vi "Handle Transmission.vi"(8 "error in (no error)":errorcluster, 11 "Stuffed Data":string) -> (0 "error out":errorcluster, 2 "Transmission valid?":bool, 3 "Transmission":string)   [LabVIEW 2015, in "LSR Transmission.lvlib"]
uses:
  LSR Transmission.lvlib
panel:
  out "Dropped Frames":i32
  out "Packets Left":i32
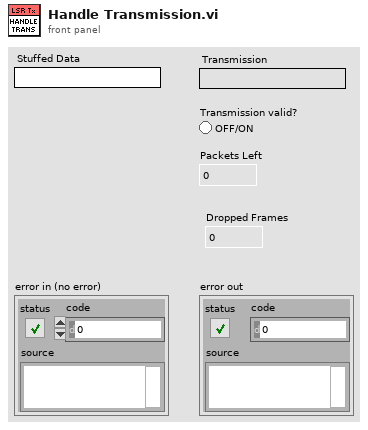
[diagram p1: front panel]
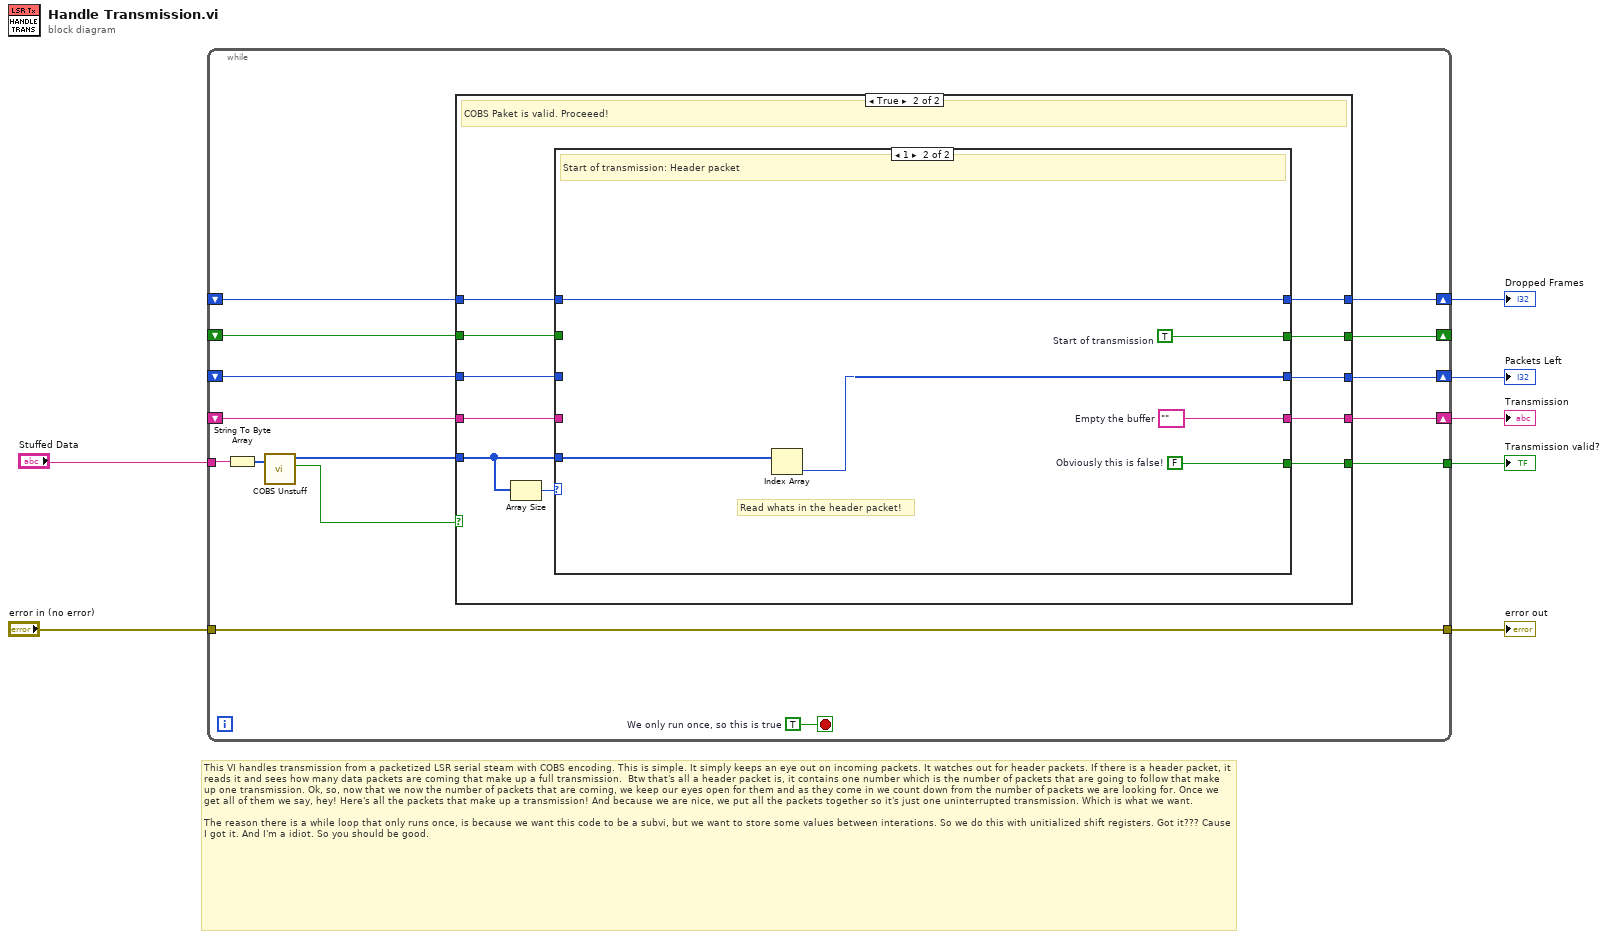
[diagram p0: block diagram]
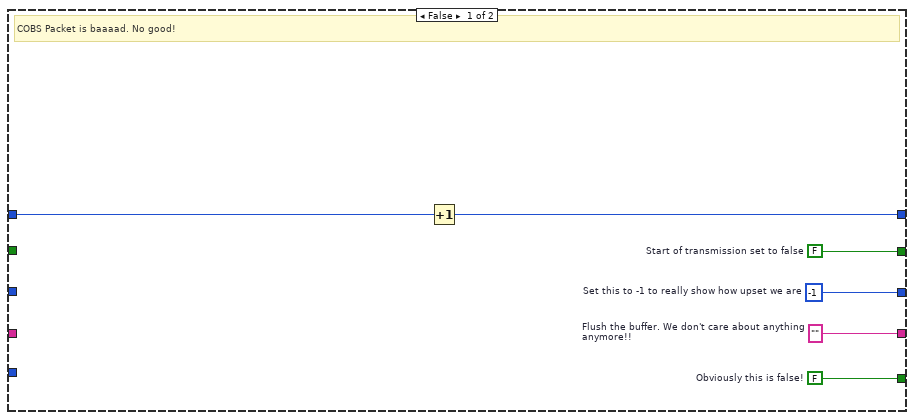
[diagram p2: hidden frame]
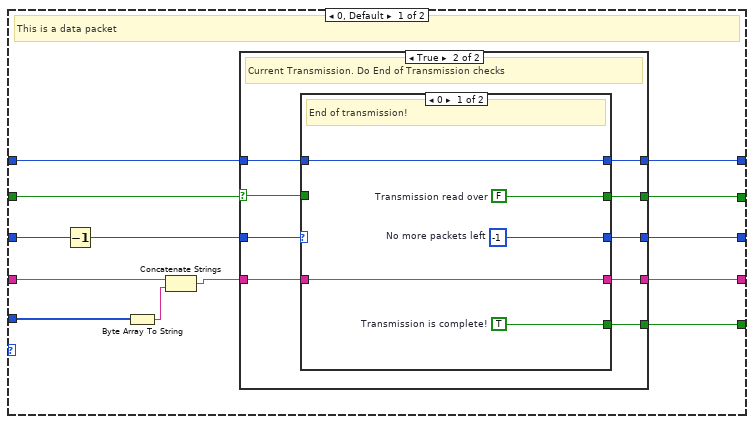
[diagram p3: hidden frame]
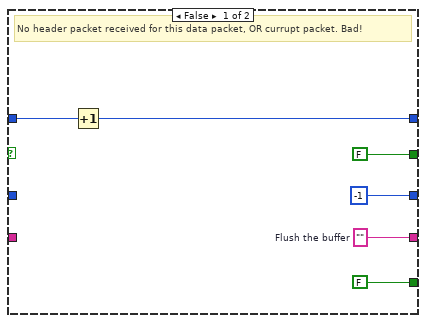
[diagram p4: hidden frame]
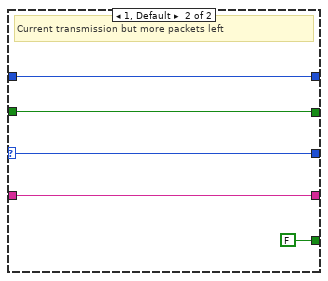
[diagram p5: hidden frame]
diagram:
  # "This VI handles transmission from a packetized LSR serial steam with COBS encoding. This is simple. It simply keeps an eye out on incoming packets. It watches out for header packets. If there is a header packet, it reads it and sees how many data packets are coming that make up a full transmission.  Btw that's all a header packet is, it contains one number which is the number of packets that are going to follow that make up one transmission. Ok, so, now that we now the number of packets that are coming, we keep our eyes open for them and as they come in we count down from the number of packets we are looking for. Once we get all of them we say, hey! Here's all the packets that make up a transmission! And because we are nice, we put all the packets together so it's just one uninterrupted transmission. Which is what we want. \n\nThe reason there is a while loop that only runs once, is because we want this code to be a subvi, but we want to store some values between interations. So we do this with unitialized shift registers. Got it??? Cause I got it. And I'm a idiot. So you should be good."
  n1 = while {
    tunnel: "Stuffed Data" -> [w10]
    shift-right: [w17] -> _
    shift-left: _ -> [w18]
    tunnel: [w16] -> w4
    shift-right: [w22] -> w2
    shift-left: _ -> [w20]
    shift-right: [w19] -> w3
    shift-left: _ -> [w21]
    tunnel: "error in (no error)" -> [w15]
    tunnel: [w15] -> w6
    shift-right: [w12] -> w1
    shift-left: _ -> [w13]
    stop <- w14 stop-if-true
    w14 = TRUE  # We only run once, so this is true
    n2 = String To Byte Array(string=w10) -> (unsigned byte array=w11:u8[])
    n3 = call "COBS Unstuff.vi"("Stuffed data in"=w11) -> ("Valid?"=w8:bool, "Unstuffed Data"=w9:u8[])  [unwired: 8 in, 1 out]
    n4 = case shown="True" w8 {
      tunnel: [w24 w39] -> w22
      tunnel: w21 -> [_ w38]
      tunnel: w20 -> [_ w37]
      tunnel: [w25 w36] -> w19
      tunnel: w18 -> [_ w35]
      tunnel: [w26 w34] -> w17
      tunnel: [w23 w33] -> w16
      tunnel: w13 -> [w28 w32]
      tunnel: [w27 w31] -> w12
      tunnel: w9 -> [_ w29]
      frame False {
        w23 = FALSE  # Obviously this is false!
        w24 = ""  # Flush the buffer. We don't care about anything anymore!!
        w25 = -1  # Set this to -1 to really show how upset we are
        w26 = FALSE  # Start of transmission set to false
        # "COBS Packet is baaaad. No good!"
        n5 = Increment(x=w28) -> (x+1=w27:i32)
      }
      frame True {
        # "COBS Paket is valid. Proceeed!"
        n6 = Array Size(array=w29) -> (size(s)=w30:i32)
        n7 = case shown="1" w30 {
          tunnel: [w47 w83] -> w39
          tunnel: w37 -> [w52 _]
          tunnel: [w49 w82] -> w36
          tunnel: w38 -> [w51 _]
          tunnel: w35 -> [w40 _]
          tunnel: [w45 w81] -> w34
          tunnel: [w44 w80] -> w33
          tunnel: w32 -> [w43 w78]
          tunnel: [w42 w78] -> w31
          tunnel: w29 -> [w41 w79]
          frame 0, Default {
            # "This is a data packet"
            n8 = Decrement(x=w51) -> (x-1=w48:i32)
            n9 = Byte Array To String(unsigned byte array=w41) -> (string=w50:string)
            n10 = Concatenate Strings(w52, w50) -> (w46:string)
            n11 = case shown="True" w40 {
              selector: w40 -> [_ w65]
              tunnel: [-1 ("No more packets left") w63] -> w49
              tunnel: w48 -> [_ w66]
              tunnel: [w55 w62] -> w47
              tunnel: w46 -> [_ w67]
              tunnel: [FALSE ("Transmission read over") w64] -> w45
              tunnel: [FALSE w61] -> w44
              tunnel: w43 -> [w57 w59]
              tunnel: [w56 w60] -> w42
              frame False {
                w55 = ""  # Flush the buffer
                # "No header packet received for this data packet, OR currupt packet. Bad!"
                n12 = Increment(x=w57) -> (x+1=w56:i32)
              }
              frame True {
                # "Current Transmission. Do End of Transmission checks"
                n13 = case shown="0" w66 {
                  selector: w66 -> [_ w76]
                  tunnel: w67 -> [w70 w75]
                  tunnel: w65 -> [_ w77]
                  tunnel: [w72 w77] -> w64
                  tunnel: [w71 w76] -> w63
                  tunnel: [w70 w75] -> w62
                  tunnel: [w69 FALSE] -> w61
                  tunnel: [w68 w73] -> w60
                  tunnel: w59 -> [w68 w73]
                  frame 0 {
                    w69 = TRUE  # Transmission is complete!
                    w71 = -1  # No more packets left
                    w72 = FALSE  # Transmission read over
                    # "End of transmission!"
                  }
                  frame 1, Default {
                    # "Current transmission but more packets left"
                  }
                }
              }
            }
          }
          frame 1 {
            w80 = FALSE  # Obviously this is false!
            w81 = TRUE  # Start of transmission
            w83 = ""  # Empty the buffer
            # "Read whats in the header packet!"
            # "Start of transmission: Header packet"
            n14 = Index Array(array=w79) -> (element=w82:u8)  [unwired: 1 in]
          }
        }
      }
    }
  }
  "error out" <- w6
  "Transmission valid?" <- w4
  "Packets Left" <- w3
  "Transmission" <- w2
  "Dropped Frames" <- w1
